vi "Read_Ch_data_file.vi"(5 "Present Channels only":bool=TRUE, 6 "Start of read offset (chars.: 0)":i64, 7 "Present Channels":string[](array[string]), 8 "Output":enum16{"All Ch data", "The last few rows"}(ring), 9 "Filename":path) -> (0 "Merged?":bool, 1 "Channel Values":string[][](array[string]), 2 "Merged Channels":string[](array[string]), 3 "exists?":bool=TRUE, 4 "Offset from File End":i64)   [LabVIEW 2020]
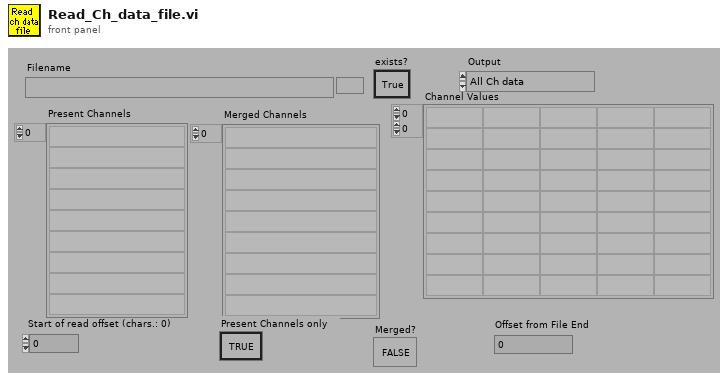
[diagram p1: front panel]
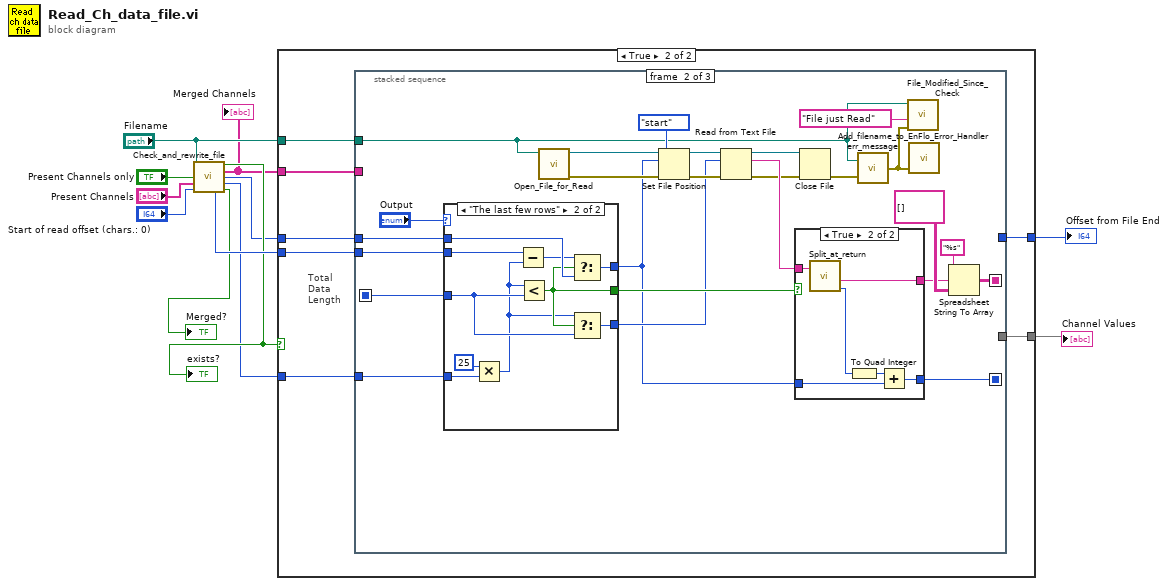
[diagram p0: block diagram]
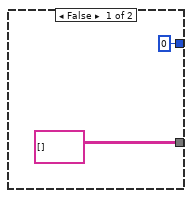
[diagram p2: hidden frame]
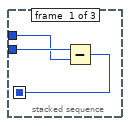
[diagram p3: hidden frame]
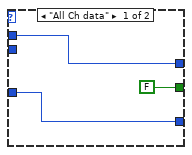
[diagram p5: hidden frame]
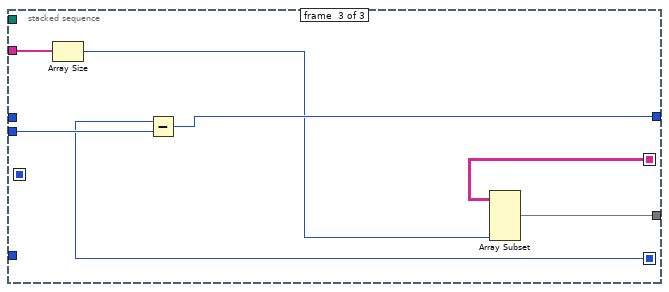
[diagram p6: hidden frame]
diagram:
  n1 = call "Check_and_rewrite_file.vi"("Filename"="Filename", "Present Channels only"="Present Channels only", "Present Channels"="Present Channels", "Start of read offset (chars.: 0)"="Start of read offset (chars.: 0)") -> ("exists?"=w6:bool, "Merged Channels"=w1:string[], "Start of data (bytes)"=w4:i64, "No of bytes/row (approx)"=w5:i64, "Current file size (bytes)"=w7:i64, "Merged?"=→"Merged?":bool)  [unwired: 6 out]
  "exists?" <- w6
  "Merged Channels" <- w1
  n2 = case shown="True" w6 {
    tunnel: [string[][] [] ("Channel Values") w20] -> w12
    tunnel: "Filename" -> [_ w21]
    tunnel: w7 -> [_ w19]
    tunnel: [i64 0 w18] -> w11
    tunnel: w5 -> [_ w17]
    tunnel: w4 -> [_ w16]
    tunnel: w1 -> [_ w15]
    frame False {
    }
    frame True {
      # "Total\nData\nLength"
      n3 = stacked-sequence {
        seq-local: [_ w46 _] -> [_ _ w75]
        seq-local: [w23 _ _] -> [_ w44 _]
        seq-local: [_ w39 _] -> [_ _ w71]
        tunnel: w21 -> [_ w27 _]
        tunnel: [_ _ w72] -> w20
        tunnel: w19 -> [w24 w45 w76]
        tunnel: [_ _ w77] -> w18
        tunnel: w17 -> [_ w41 _]
        tunnel: w16 -> [w22 w40 _]
        tunnel: w15 -> [_ _ w74]
        frame #0 {
          n4 = Subtract(x=w24, y=w22) -> (x-y=w23:i64)
        }
        frame #1 {
          n5 = case shown="\"The last few rows\"" "Output" {
            tunnel: w40 -> [w60 w68]
            tunnel: [w60 w64] -> w31
            tunnel: [w58 w65] -> w32
            tunnel: w45 -> [_ w63]
            tunnel: [FALSE w67] -> w47
            tunnel: w41 -> [_ w69]
            tunnel: w44 -> [w58 w66]
            frame "All Ch data" {
            }
            frame "The last few rows" {
              n6 = Multiply(x=i64 25 ("offset"), y=w69) -> (x*y=w62:i64)
              n7 = Subtract(x=w63, y=w62) -> (x-y=w61:i64)
              n8 = Less?(x=w62, y=w66) -> (x < y?=w67:bool)
              n9 = Select(t=w61, s=w67, f=w68) -> (s? t:f=w64:i64)
              n10 = Select(t=w62, s=w67, f=w66) -> (s? t:f=w65:i64)
            }
          }
          n11 = call "Open_File_for_Read.vi"("file path"=w27) -> ("error out"=w33:errorcluster, "refnum"=w34:refnum<file>)  [unwired: 1 in, 8 out]
          n12 = Set File Position(offset (in bytes) (0)=w31, refnum=w34, from (0:start)=enum16{"start", "end", "current"}."start", error in=w33) -> (refnum out=w37:refnum<file>, error out=w36:errorcluster)
          n13 = Read from Text File(file (use dialog)=w37, count=w32, error in=w36) -> (refnum out=w28:refnum<file>, text=w30:string, error out=w29:errorcluster)  [unwired: 1 in, 1 out]
          n14 = case shown="True" w47 {
            tunnel: w30 -> [w51 w54]
            tunnel: [w51 w55] -> w42
            tunnel: w31 -> [w50 w57]
            tunnel: [w50 w56] -> w46
            frame False {
            }
            frame True {
              n15 = call "Split_at_return.vi"("String"=w54) -> ("after substring"=w55:string, "offset past match"=w53:i32)  [unwired: 1 in, 2 out]
              n16 = To Quad Integer(1:w53) -> (0:w52:i64)
              n17 = Add(x=w52, y=w57) -> (x+y=w56:i64)
            }
          }
          n18 = Close File(refnum=w28, error in=w29) -> (error out=w38:errorcluster)  [unwired: 1 out]
          n19 = call "Add_filename_to_err_message.vi"("error in (no error)"=w38, "Path"=w27) -> ("error out"=w25:errorcluster)
          n20 = call "File_Modified_Since_Check.vi"("error in"=w25, "mode"="File just Read", "File Path"=w27) -> ()  [unwired: 5 in, 2 out]
          n21 = call "EnFlo_Error_Handler.vi"("error in (no error)"=w25) -> ()  [unwired: 2 in, 3 out]
          n22 = Spreadsheet String To Array(format string="%s", spreadsheet string=w42, array type (2D Dbl)=string[][] [] ("Channel Values")) -> (array=w39:string[][])  [unwired: 1 out]
        }
        frame #2 {
          n23 = Array Size(array=w74) -> (size(s)=w73:i32)
          n24 = Subtract(x=w75, y=w76) -> (x-y=w77:i64)
          n25 = Array Subset(array=w71, length (col)=w73) -> (w72:string[][])  [unwired: 3 in]
        }
      }
    }
  }
  "Channel Values" <- w12
  "Offset from File End" <- w11
